vi "FGV Min_Value.vi"(5 "Extrem_Value":T1, 9 "action":enum16{"set", "get"}(ring)) -> (6 "Extrem_Value 2":T1)   [LabVIEW 2014, in "FH 55.lvlib"]
doc: "In dieser FGV wird die ausgewählte Extremwertausgabe gespeichert:\n keine Ausgebe der Extremwerte\n nur Max-Werte\n Max und Min-Werte\n\n\nIn this FGV the selected output of extrem value is stored:\n no output of extreme values\n only Max values\n Max and Min values"
uses:
  FH 55.lvlib
  TypeDef/Value_String.ctl
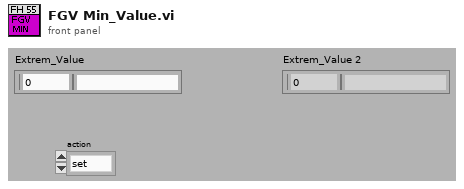
[diagram p1: front panel]
types:
  T1 = typedef "FH 55.lvlib/Value_String.ctl" = cluster{"Numeric":dbl, "String":string}
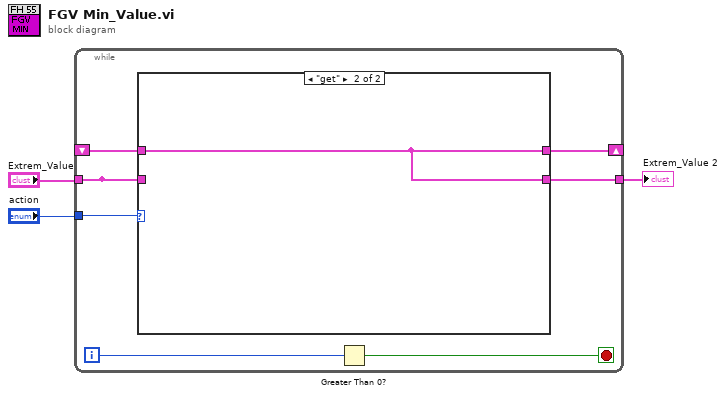
[diagram p0: block diagram]
diagram:
  n1 = while {
    tunnel: "Extrem_Value" -> [w9]
    tunnel: [w9] -> _
    shift-right: [w7] -> _
    shift-left: _ -> [w10]
    tunnel: [w8] -> w1
    tunnel: "action" -> [w4]
    i -> [w6]
    stop <- w5 stop-if-true
    n2 = case shown="\"get\"" w4 {
      tunnel: w10 -> [_ w12]
      tunnel: w9 -> [w11 _]
      tunnel: [w11 w12] -> w8
      tunnel: [w11 w12] -> w7
      frame "set", Default {
      }
      frame "get" {
      }
    }
    n3 = Greater Than 0?(x=w6) -> (x > 0?=w5:bool)
  }
  "Extrem_Value 2" <- w1
